vi "HEWH Find Non Draw.vi"(10 "Test Data -Start to End":string[][](array[string]), 11 "Draw Index":i32[][](array[numeric])) -> (3 "Non Draw Index":i32[][](array[numeric]))   [LabVIEW 2023]
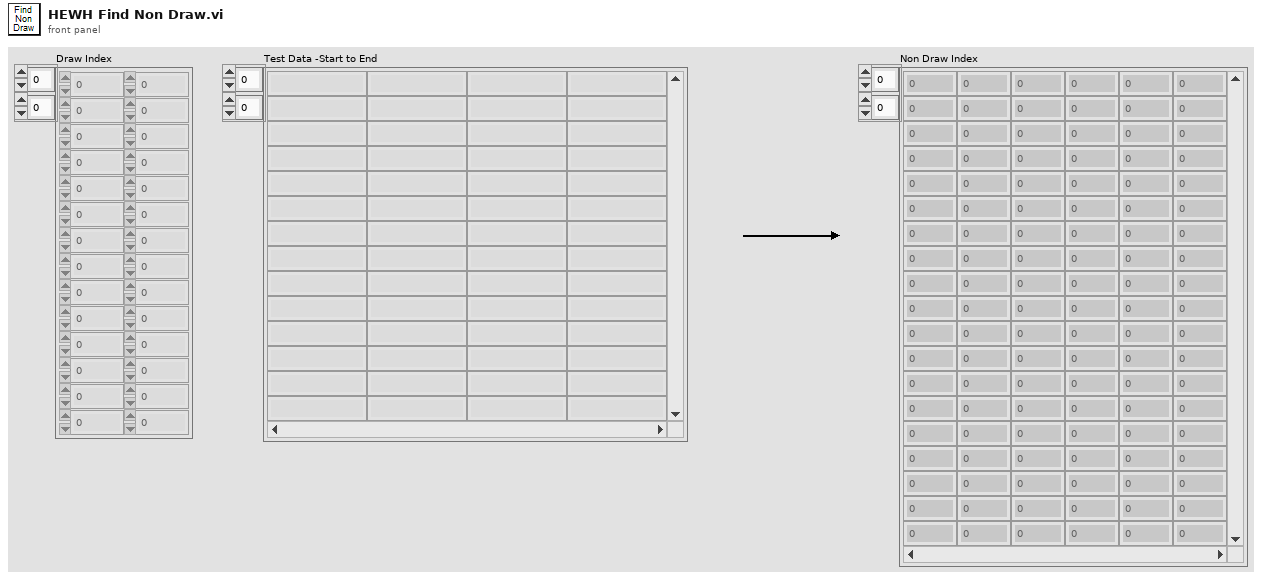
[diagram p1: front panel]
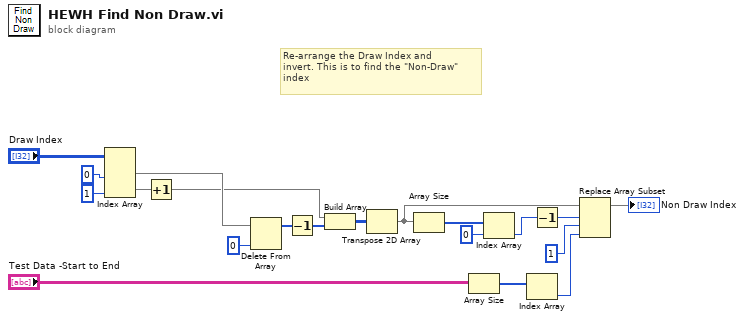
[diagram p0: block diagram]
diagram:
  # "Re-arrange the Draw Index and \ninvert. This is to find the \"Non-Draw\" \nindex"
  n1 = Index Array(array="Draw Index", index (col) #1=0 ("disabled index (col)"), index (col) #2=1 ("index (col)")) -> (element #1=w14:i32[], element #2=w9:i32[])  [unwired: 2 in]
  n2 = Increment(x=w9) -> (x+1=w8:i32[])
  n3 = Delete From Array(array=w14, index=0) -> (array with subset deleted=w11:i32[])  [unwired: 1 in, 1 out]
  n4 = Decrement(x=w11) -> (x-1=w10:i32[])
  n5 = Build Array(w8, w10) -> (w12:i32[][])
  n6 = Transpose 2D Array(2D array=w12) -> (transposed array=w5:i32[][])
  n7 = Array Size(array=w5) -> (size(s)=w7:i32[])
  n8 = Array Size(array="Test Data -Start to End") -> (size(s)=w18:i32[])
  n9 = Index Array(array=w7, index=0) -> (element=w3:i32)
  n10 = Index Array(array=w18) -> (element=w19:i32)  [unwired: 1 in]
  n11 = Decrement(x=w3) -> (x-1=w2:i32)
  n12 = Replace Array Subset(array=w5, new element=w19, index (row)=w2, index (col)=1 ("disabled index (col)")) -> (→"Non Draw Index":i32[][])
